vi "Finish.vi"(4 "error in (no error)":errorcluster) -> (0 "error out":errorcluster)   [LabVIEW 2013]
doc: "This VI is called just before exiting. It is expected to close I/O refnum, save collected data, etc."
uses:
  <vilib>/Rock Robotics/WPI/Joystick/WPI_JoystickGetSetRefNum.vi
  <vilib>/Rock Robotics/WPI/RobotDrive/WPI_RobotDriveGetSetRefNum.vi
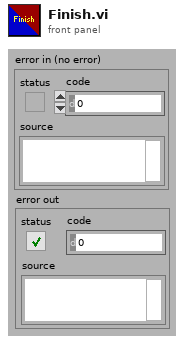
[diagram p1: front panel]
types:
  T1 = typedef "WPI_JoystickDevRef.ctl" = cluster{"Device":T2}
  T2 = typedef "WPI_JoystickDeviceEnum.ctl" = enum16{"USB 1", "USB 2", "USB 3", "USB 4", "Kinect 1", "Kinect 2"}
  T3 = typedef "WPI_RelayDevRef.ctl" = cluster{"DevStatus":errorcluster, "Relay Channel":T4, "Digital Module":T5, "Relay Direction":T6}
  T4 = typedef "FPGA_DIORelayChannel.ctl" = enum8{"Relay 1", "Relay 2", "Relay 3", "Relay 4", "Relay 5", "Relay 6", "Relay 7", "Relay 8", "Invalid"}
  T5 = typedef "FPGA_TypedefDigitalModule.ctl" = enum16{"Digital Module 1", "Digital Module 2"}
  T6 = typedef "WPI_RelayDirection.ctl" = enum16{"Both directions", "Forward only", "Reverse only"}
  T7 = typedef "WPI_RobotDriveDevRef.ctl" = cluster{"DevStatus":errorcluster, "Motors[]":T8[], "Square Inputs":bool, "Max Output":dbl, "Isochronous":bool}
  T8 = typedef "WPI_MotorControlDeviceRef.ctl" = cluster{"DeviceStatus":errorcluster, "Type":enum16{"PWM", "CAN"}, "PWM":cluster{"Digital Module":T5, "PWM Channel":T9, "DeadBand":T10}, "CAN":cluster{"Device Number":u8, "Control Mode":T11, "Semaphore":T12, "Max Vout":dbl}, "Invert":bool, "TransformRef":T13, "InvTransformRef":T13}
  T9 = typedef "FPGA_DIOPWMChannel.ctl" = enum8{"PWM 1", "PWM 2", "PWM 3", "PWM 4", "PWM 5", "PWM 6", "PWM 7", "PWM 8", "PWM 9", "PWM 10", "Invalid"}
  T10 = typedef "WPI_PWMDeadband.ctl" = cluster{"Name":string, "maxPositivePwm":i32, "minPositivePwm":i32, "centerPwm":i32, "maxNegativePwm":i32, "minNegativePwm":i32, "angularRange":u16}
  T11 = typedef "WPI_CANJaguar_ControlMode.ctl" = enum8{"Percent VBus", "Current", "Speed", "Position", "Voltage"}
  T12 = typedef "Semaphore RefNum" = refnum<k1>
  T13 = typedef "WPI_PWMTransform_ConPane.ctl" = refnum<vi>
  T14 = typedef "WPI_CameraDevRef.ctl" = cluster{"Camera Address":string, "CameraStatus":errorcluster, "Acquire Image Notifier":refnum<notifier>}
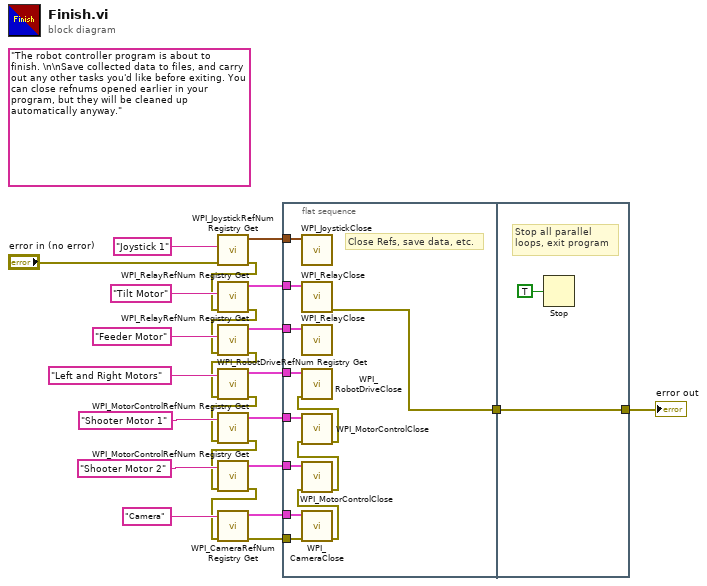
[diagram p0: block diagram]
diagram:
  (unwired) "The robot controller program is about to finish. \n\nSave collected data to files, and carry out any other tasks you'd like before exiting. You can close refnums opened earlier in your program, but they will be cleaned up automatically anyway."
  n1 = call <vilib>:"WPI_JoystickRefNum Registry Get.vi"("error in (no error)"="error in (no error)", "refnum name"="Joystick 1") -> ("error out"=w10:errorcluster, "JoystickDevRef"=w19:T1)  [unwired: 8 out]
  n2 = call <vilib>:"WPI_RelayRefNum Registry Get.vi"("error in (no error)"=w10, "refnum name"="Tilt Motor") -> ("error out"=w11:errorcluster, "RelayDevRef"=w18:T3)  [unwired: 8 in]
  n3 = call <vilib>:"WPI_RelayRefNum Registry Get.vi"("error in (no error)"=w11, "refnum name"="Feeder Motor") -> ("error out"=w7:errorcluster, "RelayDevRef"=w13:T3)  [unwired: 8 in]
  n4 = call <vilib>:"WPI_RobotDriveRefNum Registry Get.vi"("error in (no error)"=w7, "refnum name"="Left and Right Motors") -> ("error out"=w6:errorcluster, "RobotDriveDevRef"=w17:T7)  [unwired: 8 out]
  n5 = call <vilib>:"WPI_MotorControlRefNum Registry Get.vi"("error in (no error)"=w6, "refnum name"="Shooter Motor 1") -> ("error out"=w5:errorcluster, "MotorControlDevRef"=w9:T8)  [unwired: 8 in]
  n6 = call <vilib>:"WPI_MotorControlRefNum Registry Get.vi"("error in (no error)"=w5, "refnum name"="Shooter Motor 2") -> ("error out"=w4:errorcluster, "MotorControlDevRef"=w16:T8)  [unwired: 8 in]
  n7 = call <vilib>:"WPI_CameraRefNum Registry Get.vi"("error in (no error)"=w4, "refnum name"="Camera") -> ("error out"=w3:errorcluster, "CameraDevRef"=w15:T14)  [unwired: 8 out]
  n8 = flat-sequence {
    tunnel: w19 -> [w36]
    tunnel: w18 -> [w35]
    tunnel: w17 -> [w34]
    tunnel: w16 -> [w33]
    tunnel: w15 -> [w32]
    tunnel: w13 -> [w31]
    tunnel: w9 -> [w30]
    tunnel: w3 -> [w27]
    tunnel: [w25] -> w2
    tunnel: [w37] -> w1
    tunnel: w2 -> [w37]
    frame #0 {
      # "Close Refs, save data, etc."
      n9 = call <vilib>:"WPI_JoystickClose.vi"("JoystickDevRef"=w36) -> ()  [unwired: 11 out]
      n10 = call <vilib>:"WPI_RelayClose.vi"("RelayDevRef"=w35) -> ("error out"=w25:errorcluster)  [unwired: 10 in]
      n11 = call <vilib>:"WPI_RelayClose.vi"("RelayDevRef"=w31) -> ()  [unwired: 10 in, 1 out]
      n12 = call <vilib>:"WPI_CameraClose.vi"("error in (no error)"=w27, "CameraDevRef"=w32) -> ("error out"=w26:errorcluster)  [unwired: 9 out]
      n13 = call <vilib>:"WPI_MotorControlClose.vi"("error in (no error)"=w26, "MotorControlDevRef"=w33) -> ("error out"=w29:errorcluster)  [unwired: 9 in]
      n14 = call <vilib>:"WPI_MotorControlClose.vi"("error in (no error)"=w29, "MotorControlDevRef"=w30) -> ("error out"=w28:errorcluster)  [unwired: 9 in]
      n15 = call <vilib>:"WPI_RobotDriveClose.vi"("error in (no error)"=w28, "RobotDriveDevRef"=w34) -> ()  [unwired: 10 out]
    }
    frame #1 {
      # "Stop all parallel\nloops, exit program"
      n16 = Stop(stop? (T)=TRUE ("Quit")) -> ()
    }
  }
  "error out" <- w1
